vi "Boxes_Separated.vi"(0 "Box 1":T1=[{"Max"=16000.0, "Min"=14000.0}, {"Max"=1000.0, "Min"=-1000.0}, {"Max"=700.0, "Min"=0.0}] {"Min" format="%#.1f"; "Max" format="%#.1f"}, 1 "Box 2":T1=[{"Max"=16000.0, "Min"=14000.0}, {"Max"=1000.0, "Min"=-1000.0}, {"Max"=700.0, "Min"=0.0}] {"Min" format="%#.1f"; "Max" format="%#.1f"}) -> (2 "Box Separated":bool, 3 "Error String":string, 4 "Separation Distance":sgl format="%.2f")   [LabVIEW 2014]
uses:
  Box_size.ctl
panel:
  # "X                           Y                          Z"
  # "X                           Y                          Z"
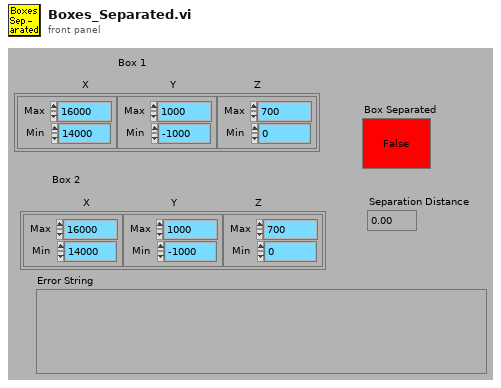
[diagram p1: front panel]
types:
  T1 = typedef "Box_size.ctl" = cluster{"Max":sgl, "Min":sgl}[]
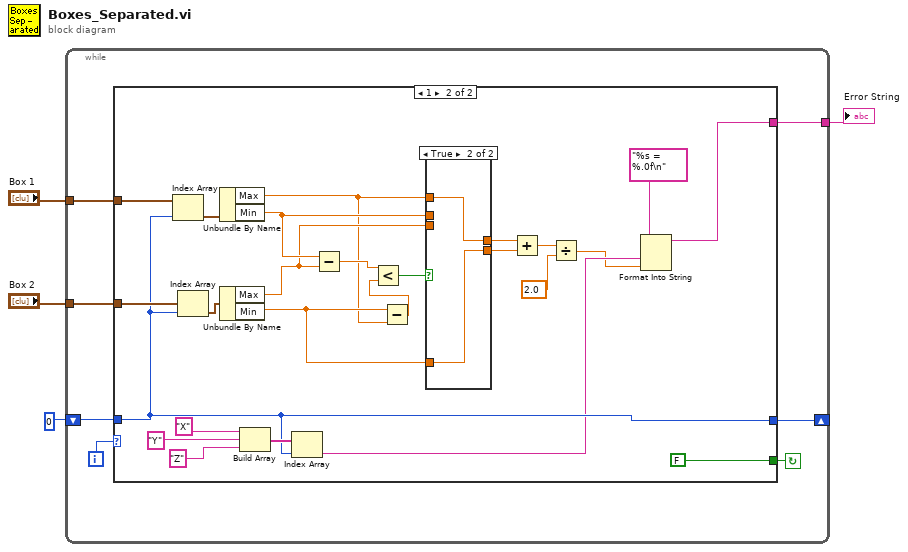
[diagram p0: block diagram]
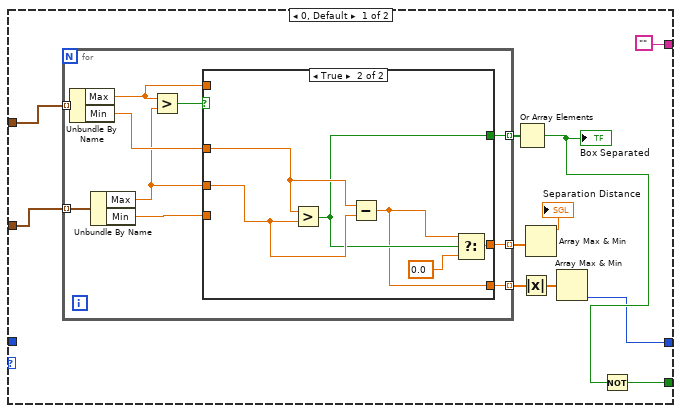
[diagram p2: hidden frame]
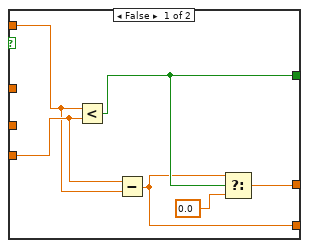
[diagram p3: hidden frame]
diagram:
  n1 = while {
    tunnel: [w5] -> w1
    shift-left: 0 -> [w8]
    shift-right: [w7] -> _
    tunnel: "Box 2" -> [w10]
    tunnel: "Box 1" -> [w11]
    i -> [w6]
    stop <- w9 continue-if-true
    n2 = case shown="1" w6 {
      tunnel: w11 -> [w18 w69]
      tunnel: w10 -> [w17 w68]
      tunnel: [w22 FALSE] -> w9
      tunnel: w8 -> [_ w49]
      tunnel: [w13 w49] -> w7
      tunnel: ["" w45] -> w5
      frame 0, Default {
        n3 = for {
          tunnel: w18 -> [w32] mode=indexing
          tunnel: [w26] -> w19 mode=indexing
          tunnel: [w25] -> w20 mode=indexing
          tunnel: [w24] -> w15 mode=indexing
          tunnel: w17 -> [w23] mode=indexing
          n4 = Unbundle By Name(w32) -> ("Max"=w28:sgl, "Min"=w30:sgl)
          n5 = Unbundle By Name(w23) -> ("Max"=w29:sgl, "Min"=w27:sgl)
          n6 = Greater?(x=w28, y=w29) -> (0:w31:bool)
          n7 = case shown="True" w31 {
            tunnel: w30 -> [_ w44]
            tunnel: w29 -> [_ w43]
            tunnel: w28 -> [w37 _]
            tunnel: w27 -> [w38 _]
            tunnel: [w36 w41] -> w26
            tunnel: [w34 w40] -> w25
            tunnel: [w33 w39] -> w24
            frame False {
              n8 = Less?(x=w37, y=w38) -> (x < y?=w36:bool)
              n9 = Subtract(x=w38, y=w37) -> (x-y=w33:sgl)
              n10 = Select(t=w33, s=w36, f=0.0) -> (s? t:f=w34:dbl)
            }
            frame True {
              n11 = Greater?(x=w44, y=w43) -> (0:w41:bool)
              n12 = Subtract(x=w44, y=w43) -> (x-y=w39:sgl)
              n13 = Select(t=w39, s=w41, f=0.0) -> (s? t:f=w40:dbl)
            }
          }
        }
        n14 = Or Array Elements(Boolean array=w19) -> (logical OR=w16:bool)
        "Box Separated" <- w16
        n15 = Absolute Value(x=w15) -> (abs(x)=w14:sgl[])
        n16 = Array Max & Min(array=w20) -> (max value=→"Separation Distance":dbl)  [unwired: 3 out]
        n17 = Array Max & Min(array=w14) -> (min index (indices)=w13:i32)  [unwired: 3 out]
        n18 = Not(x=w16) -> (.not. x?=w22:bool)
      }
      frame 1 {
        n19 = Index Array(array=w69, index=w49) -> (element=w66:cluster{"Max":sgl, "Min":sgl})
        n20 = Index Array(array=w68, index=w49) -> (element=w67:cluster{"Max":sgl, "Min":sgl})
        n21 = Unbundle By Name(w66) -> ("Max"=w54:sgl, "Min"=w61:sgl)
        n22 = Unbundle By Name(w67) -> ("Max"=w60:sgl, "Min"=w55:sgl)
        n23 = Build Array("X", "Y", "Z") -> (w50:string[])
        n24 = Index Array(array=w50, index=w49) -> (element=w47:string)
        n25 = Subtract(x=w61, y=w60) -> (x-y=w64:sgl)
        n26 = Subtract(x=w55, y=w54) -> (x-y=w63:sgl)
        n27 = Less?(x=w64, y=w63) -> (x < y?=w62:bool)
        n28 = case shown="True" w62 {
          tunnel: w61 -> [w71 _]
          tunnel: w60 -> [w70 _]
          tunnel: [w71 w72] -> w57
          tunnel: [w70 w73] -> w56
          tunnel: w55 -> [_ w73]
          tunnel: w54 -> [_ w72]
          frame False {
          }
          frame True {
          }
        }
        n29 = Add(x=w57, y=w56) -> (x+y=w59:sgl)
        n30 = Divide(x=w59, y=sgl 2.0) -> (x/y=w46:sgl)
        n31 = Format Into String(format string="%s = %.0f\n" ("Format String"), w47, w46) -> (resulting string=w45:string)  [unwired: 2 in, 1 out]
      }
    }
  }
  "Error String" <- w1
